vi "3458A Initialize Virtual Channels.vi"(8 "error in":errorcluster, 10 "reset instruments (False)":bool, 11 "digitizer in":T1 {"channels"."Range [Vpk]" min=0.0}) -> (0 "error out":errorcluster, 1 "awg idn string":string, 2 "dmm(s) idn strings":string[](array[string]), 3 "digitizer out":T1 {"channels"."Range [Vpk]" min=0.0}, 4 "sync unit idn string":string)   [LabVIEW 2013, in "3458A Virtual Digitizer.lvlib"]
doc: "Call this to open all intruments related to the digitizing DMMs system.\n1) Opens all 3458A channels.\n2) If needed for selected mode, opens counter for measurement of two channels time shift (used for 3458A with synchronized clocks).\n3) If needed for selected mode, opens AWG."
uses:
  3458A Virtual Digitizer.lvlib
  3458A Digitizer Session.ctl
  3458A Virtual Channel Config.ctl
  Counter/Counter Session.ctl
  Counter/Counter Type.ctl
  AWG/AWG Session.ctl
  AWG/AWG Type.ctl
  3458A Sync Mode.ctl
  3458A Idn Mode.ctl
  3458A Digitizing Low Levels/Configure/Sampling Mode.ctl
  3458A Digitizing Process Options.ctl
  3458A Data Packet.ctl
  3458A Aux Record Data.ctl
  3458A Digitizing Low Levels/Configure/Level Setup.ctl
  3458A Digitizing Low Levels/Configure/First Sample Trigger.ctl
  3458A Aperture Selection Mode.ctl
  3458A Digitizing Low Levels/3458A Digitizing Low Levels.lvlib
  AWG/AWG.lvlib
  Counter/Counter.lvlib
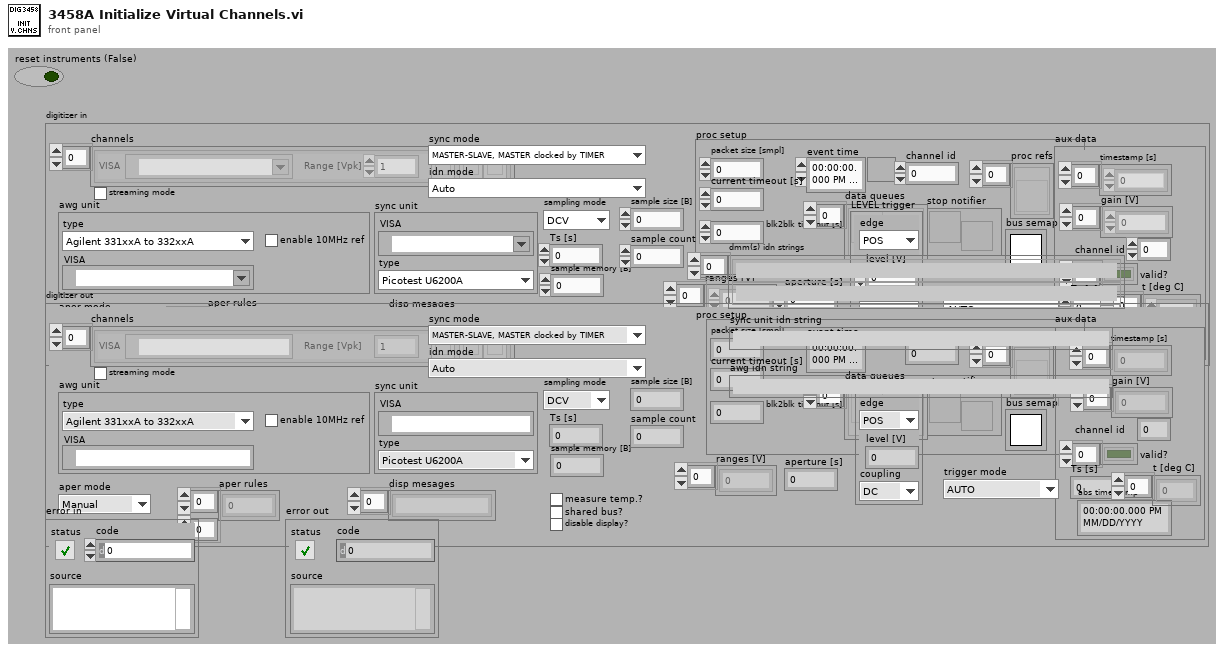
[diagram p1: front panel]
types:
  T1 = typedef "3458A Virtual Digitizer.lvlib/3458A Digitizer Session.ctl" = cluster{"channels":T2[], "sync unit":T3, "awg unit":T5, "sync mode":T7, "streaming mode":bool, "idn mode":T8, "sampling mode":T9, "Ts [s]":dbl, "sample memory [B]":i32, "proc setup":T10, "sample size [B]":i32, "sample count":i32, "aux data":T12, "ranges [V]":dbl[], "aperture [s]":dbl, "LEVEL trigger":T13, "trigger mode":T14, "measure temp.?":bool, "disp mesages":string[], "shared bus?":bool, "disable display?":bool, "aper mode":T15, "aper rules":dbl[][]}
  T2 = typedef "3458A Virtual Digitizer.lvlib/3458A Virtual Channel Config.ctl" = cluster{"VISA":refnum<visa-resource-name>, "Range [Vpk]":dbl, "btn clr":bool, "btn up":bool, "btn down":bool}
  T3 = typedef "Counter.lvlib/Counter Session.ctl" = cluster{"VISA":refnum<visa-resource-name>, "type":T4}
  T4 = typedef "Counter.lvlib/Counter Type.ctl" = enum16{"Picotest U6200A", "dummy"}
  T5 = typedef "AWG.lvlib/AWG Session.ctl" = cluster{"type":T6, "VISA":refnum<visa-resource-name>, "enable 10MHz ref":bool}
  T6 = typedef "AWG.lvlib/AWG Type.ctl" = enum16{"Agilent 331xxA to 332xxA", "Agilent 335xxA to 336xxA", "Tektronix AFG3101C", "dummy"}
  T7 = typedef "3458A Virtual Digitizer.lvlib/3458A Sync Mode.ctl" = enum16{"MASTER-SLAVE, MASTER clocked by TIMER", "MASTER-SLAVE, MASTER clocked by AWG", "ALL clocked by AWG", "MASTER-SLAVE, ALL clocked by TIMER", "ALL clocked by AWG with DFLL"}
  T8 = typedef "3458A Virtual Digitizer.lvlib/3458A Idn Mode.ctl" = enum16{"Auto", "Sequential (chn A, chn B, ...)", "From calibration string"}
  T9 = typedef "3458A Virtual Digitizer.lvlib/3458A Digitizing Low Levels.lvlib/Sampling Mode.ctl" = enum16{"DCV", "DSDC", "DSAC"}
  T10 = typedef "3458A Virtual Digitizer.lvlib/3458A Digitizing Process Options.ctl" = cluster{"channel id":i32, "packet size [smpl]":i32, "current timeout [s]":dbl, "blk2blk timeout [s]":dbl, "event time":timestamp, "stop notifier":refnum<notifier>, "data queues":refnum<queue>[], "proc refs":refnum<vi>[], "bus semaphore":T11}
  T11 = typedef "Semaphore RefNum" = refnum<k1>
  T12 = typedef "3458A Virtual Digitizer.lvlib/3458A Aux Record Data.ctl" = cluster{"channel id":i32, "valid?":bool[], "gain [V]":dbl[], "timestamp [s]":dbl[], "Ts [s]":dbl, "abs timestamp":timestamp, "t [deg C]":dbl[]}
  T13 = typedef "3458A Virtual Digitizer.lvlib/3458A Digitizing Low Levels.lvlib/Level Setup.ctl" = cluster{"edge":enum16{"POS", "NEG"}, "level [V]":dbl, "coupling":enum16{"DC", "AC"}}
  T14 = typedef "3458A Virtual Digitizer.lvlib/3458A Digitizing Low Levels.lvlib/First Sample Trigger.ctl" = enum16{"AUTO", "EXT", "SYN", "SGL", "HOLD", "LEVEL"}
  T15 = typedef "3458A Virtual Digitizer.lvlib/3458A Aperture Selection Mode.ctl" = enum16{"Manual", "Maximum", "Table"}
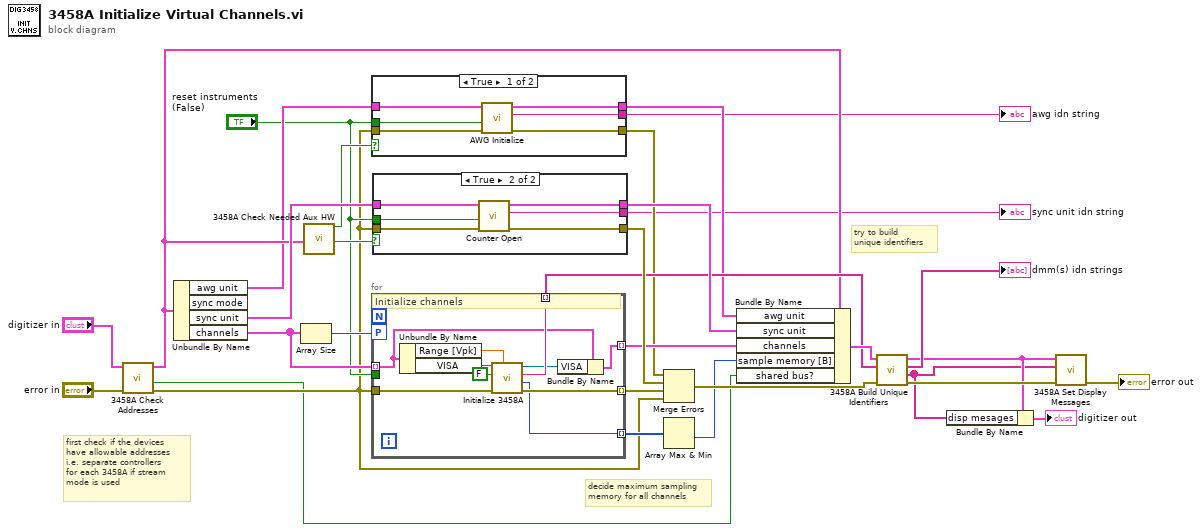
[diagram p0: block diagram]
diagram:
  # "decide maximum sampling\nmemory for all channels"
  # "try to build\nunique identifiers"
  # "first check if the devices\nhave allowable addresses\ni.e. separate controllers\nfor each 3458A if stream\nmode is used"
  n1 = call "3458A Check Addresses.vi"("error in"="error in", "digitizer session in"="digitizer in") -> ("error out"=w2:errorcluster, "some dmms shares the same controller?"=w1:bool, "digitizer session out"=w17:T1)  [unwired: 6 in, 1 out]
  n2 = Unbundle By Name(w17) -> ("awg unit"=w16:T5, "sync unit"=w28:T3, "channels"=w31:T2[])  [unwired: 1 out]
  n3 = Array Size(array=w31) -> (size(s)=w30:i32)
  n4 = call "3458A Check Needed Aux HW.vi"("digitizer session"=w17) -> ("uses AWG clocking?"=w14:bool, "uses counter?"=w15:bool)  [unwired: 13 in, 4 out]
  n5 = case shown="True" w14 {
    tunnel: w2 -> [w37 w39]
    tunnel: [w34 w39] -> w13
    tunnel: w16 -> [w36 w38]
    tunnel: [w35 w38] -> w12
    tunnel: [w33 _] -> w11
    tunnel: "reset instruments (False)" -> [w32 _]
    frame True {
      # "Initialize AWG"
      n6 = call "AWG Initialize.vi"("error in (no error)"=w37, "Reset (True)"=w32, "awg session in"=w36) -> ("error out"=w34:errorcluster, "idn string"=w33:string, "awg session out"=w35:T5)  [unwired: 6 in]
    }
    frame False {
    }
  }
  "awg idn string" <- w11
  n7 = for {
    tunnel: w2 -> [w49]
    tunnel: w31 -> [w44] mode=indexing
    workers-P: w30 -> [_]
    tunnel: [w48] -> w29 mode=indexing
    tunnel: [w43] -> w25 mode=indexing
    tunnel: [w47] -> w20 mode=indexing
    tunnel: "reset instruments (False)" -> [_]
    tunnel: [w42] -> w19 mode=indexing
    # "Initialize channels"
    n8 = Unbundle By Name(w44) -> ("Range [Vpk]"=w40:dbl, "VISA"=w46:refnum<visa-resource-name>)
    n9 = call "Initialize 3458A.vi"("range [V] (10V)"=w40, "error in (no error)"=w49, "Reset (True)"=FALSE, "VISA DMM"=w46) -> ("error out"=w48:errorcluster, "sample memory [B]"=w42:i32, "idn string"=w47:string, "VISA resource name out"=w45:refnum<visa-resource-name>)  [unwired: 4 in]
    n10 = Bundle By Name(cluster=w44, "VISA"=w45) -> (w43:T2)
  }
  n11 = case shown="True" w15 {
    tunnel: w2 -> [w50 w57]
    tunnel: w28 -> [w51 w56]
    tunnel: [w50 w54] -> w27
    tunnel: [w51 w52] -> w26
    tunnel: "reset instruments (False)" -> [_ w55]
    tunnel: [_ w53] -> w9
    frame False {
      # "Initialize AWG"
    }
    frame True {
      # "Initialize counter"
      n12 = call "Counter Open.vi"("error in"=w57, "Reset (True)"=w55, "couner session in"=w56) -> ("error out"=w54:errorcluster, "idn string"=w53:string, "counter session out"=w52:T3)  [unwired: 6 in]
    }
  }
  "sync unit idn string" <- w9
  n13 = Merge Errors(w13, w27, w29, w2) -> (w22:errorcluster)
  n14 = Array Max & Min(array=w19) -> (min value=w18:i32)  [unwired: 3 out]
  n15 = Bundle By Name(cluster=w17, "awg unit"=w12, "sync unit"=w26, "channels"=w25, "sample memory [B]"=w18, "shared bus?"=w1) -> (w21:T1)
  n16 = call "3458A Build Unique Identifiers.vi"("error in"=w22, "dmm(s) idn strings in"=w20, "digitizer session in"=w21) -> ("error out"=w8:errorcluster, "display strings"=w4:string[], "identifier strings"=→"dmm(s) idn strings":string[], "digitizer session out"=w5:T1)  [unwired: 5 in]
  n17 = Bundle By Name(cluster=w5, "disp mesages"=w4) -> (→"digitizer out":T1)
  n18 = call "3458A Set Display Messages.vi"("error in (no error)"=w8, "display strings"=w4, "digitizer session in"=w5) -> ("error out"=→"error out":errorcluster)  [unwired: 7 in, 1 out]
